vi "Report.WR.vi"(0 "Report Path":path=path "C:/Documents and Settings/Administrator/桌面", 1 "TestTime":dbl, 2 "TestRecord":T2={"name_pf"="Product_name", "name_name_ean13"="input SN", "supplier_code"="", "date"="", "time"="", "operater_code"="0", "sw_code"="", "sw_ver"="V10", "test_type"="EOL", "spare"="", "jig_code"="T001", "total_qty"="0", "field_code"="", "test_time"="NA", "test_result"="NA", "serial_number"="input SN", "TestItem"=[]}, 4 "SN":string, 5 "Result":enum16{"PASS", "FAIL", "INT.", "TOUT"}(ring)=enum."FAIL", 6 "TestTime":T1) -> (7 "OK?":bool=TRUE, 8 "TestTime?":bool, 9 "FileName":string="C:\\Documents and Settings\\Administrator\\桌面\\report\\Product_name_T001_EOL_800324.txt")   [LabVIEW 2012, in "Lib_UEL.ATE.lvlib" / "Lib_Report.lvlib"]
uses:
  Lib_Report.lvlib
panel:
  out "SystemTime":string="20121102  17:33:22 "
  # "ChangeLog\n2014-6-19: 根据UD反馈，修改栏目对齐问题。"
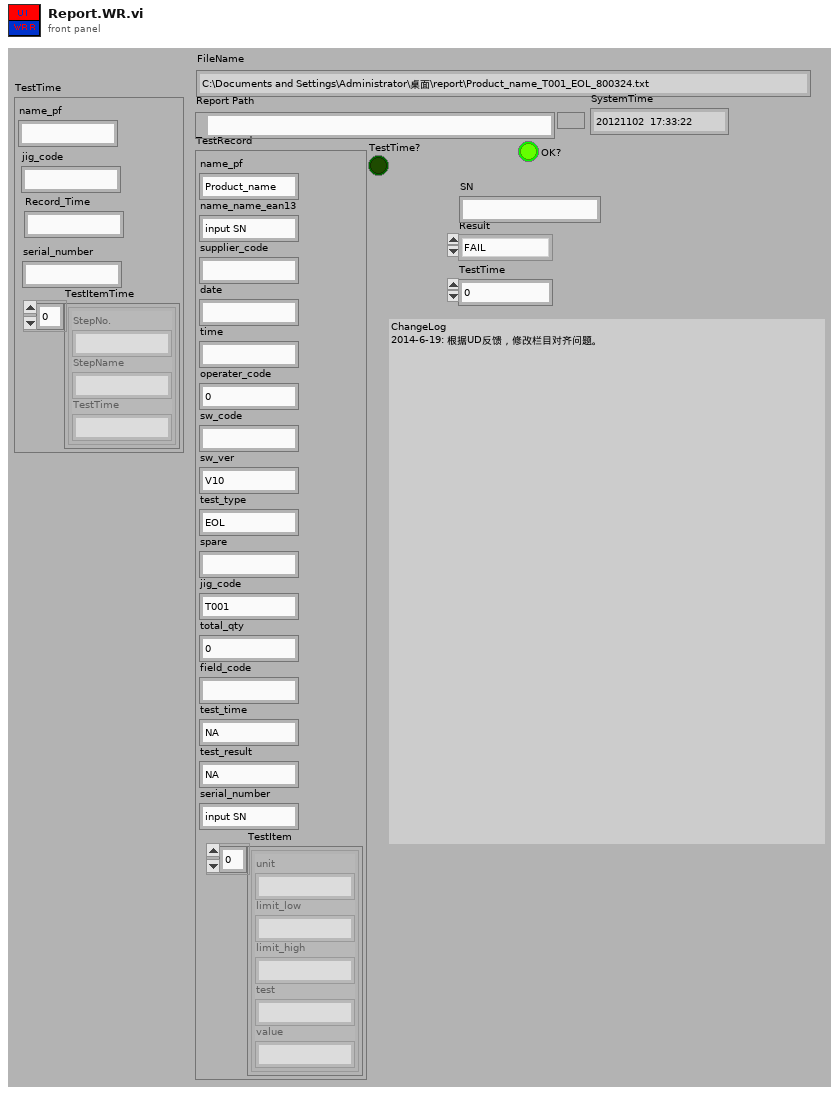
[diagram p1: front panel]
types:
  T1 = cluster{"name_pf":string, "jig_code":string, "Record_Time":string, "serial_number":string, "TestItemTime":cluster{"StepNo.":string, "StepName":string, "TestTime":string}[]}
  T2 = cluster{"name_pf":string, "name_name_ean13":string, "supplier_code":string, "date":string, "time":string, "operater_code":string, "sw_code":string, "sw_ver":string, "test_type":string, "spare":string, "jig_code":string, "total_qty":string, "field_code":string, "test_time":string, "test_result":string, "serial_number":string, "TestItem":cluster{"unit":string, "limit_low":string, "limit_high":string, "test":string, "value":string}[]}
  T3 = enum16{"open", "replace", "create", "open or create", "replace or create", "replace or create with confirmation"}
  T4 = cluster{"unit":string, "limit_low":string, "limit_high":string, "test":string, "value":string}[]
  T5 = cluster{"StepNo.":string, "StepName":string, "TestTime":string}[]
  T6 = cluster{"unit":string, "limit_low":string, "limit_high":string, "test":string, "value":string}
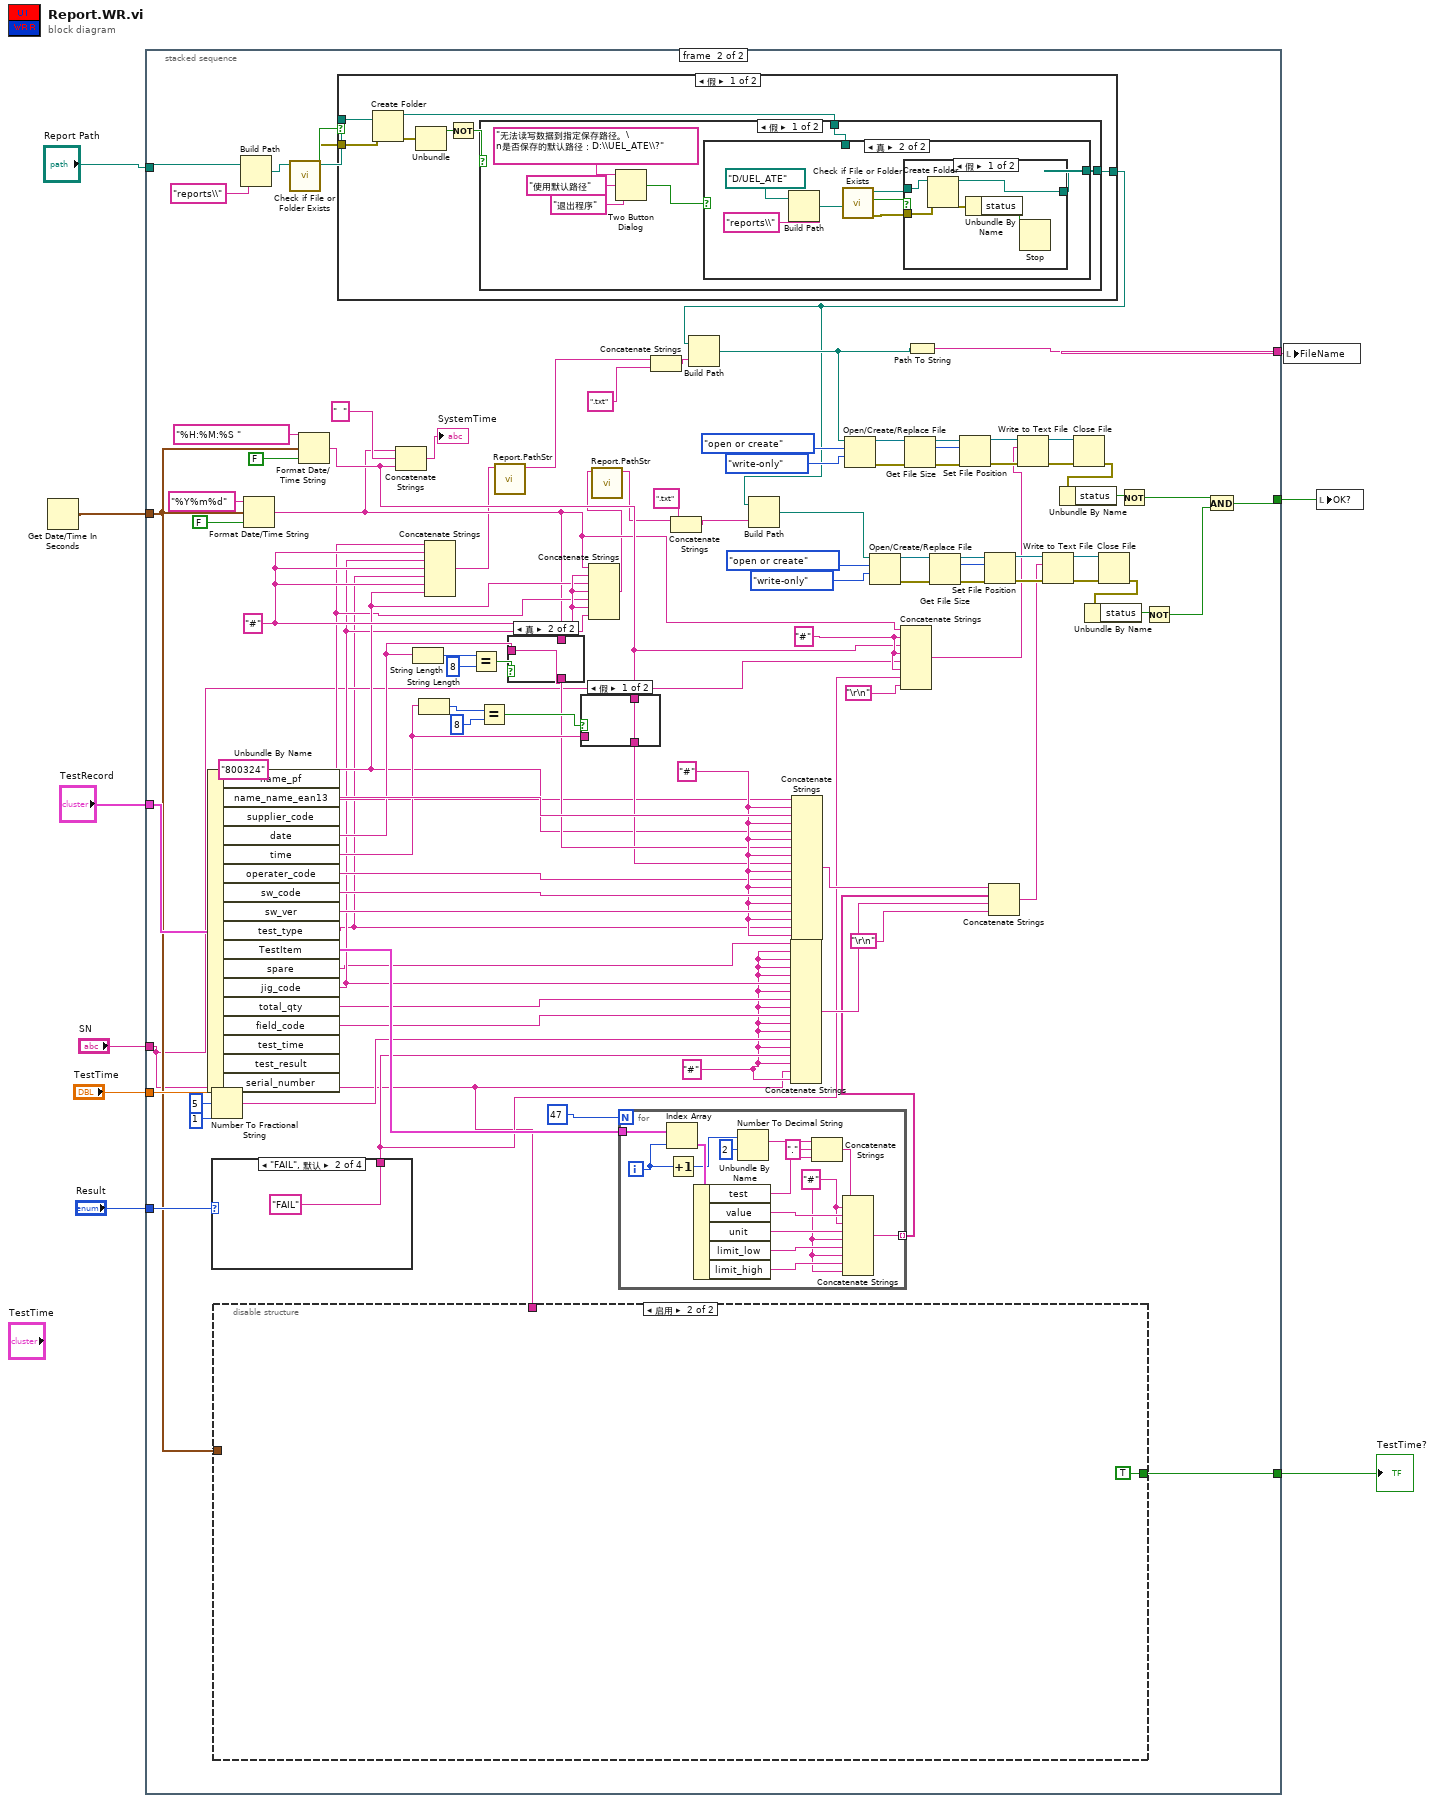
[diagram p0: block diagram]
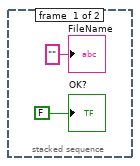
[diagram p2: hidden frame]
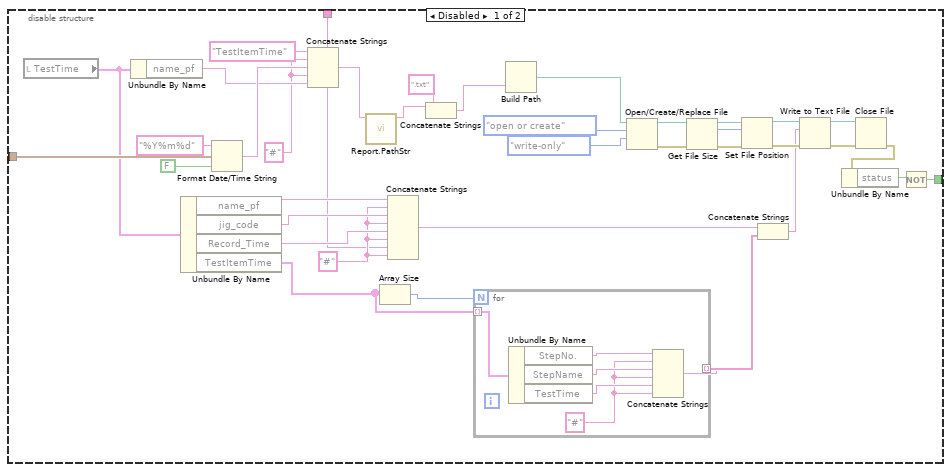
[diagram p3: hidden frame]
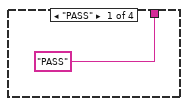
[diagram p4: hidden frame]
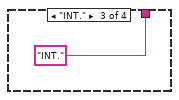
[diagram p5: hidden frame]
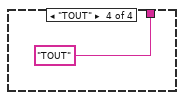
[diagram p6: hidden frame]
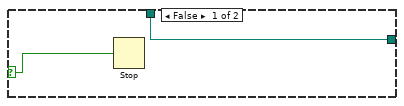
[diagram p9: hidden frame]
diagram:
  n1 = Get Date/Time In Seconds() -> (seconds since 1Jan1904=w8:timestamp)
  n2 = stacked-sequence {
    tunnel: "Report Path" -> [_ w21]
    tunnel: w8 -> [_ w15]
    tunnel: "TestRecord" -> [_ w101]
    tunnel: [_ w83] -> w6
    tunnel: [_ w29] -> w5
    tunnel: "Result" -> [_ w58]
    tunnel: "TestTime" -> [_ w57]
    tunnel: "SN" -> [_ w13]
    tunnel: [_ w14] -> w1
    frame #0 {
      "FileName" <- "" ("FileName")
      "OK?" <- FALSE ("OK?")
    }
    frame #1 {
      w33 = "#" ("字符串")
      w40 = "#" ("字符串")
      w39 = "800324" ("字符串")
      w17 = "#" ("字符串")
      w95 = "#" ("字符串")
      n3 = Unbundle By Name(w101) -> ("name_pf"=w38:string, "name_name_ean13"=w98:string, "date"=w64:string, "time"=w63:string, "operater_code"=w59:string, "sw_code"=w97:string, "sw_ver"=w96:string, "test_type"=w12:string, "TestItem"=w99:T4, "spare"=w20:string, "jig_code"=w37:string, "total_qty"=w94:string, "field_code"=w93:string)  [unwired: 4 out]
      n4 = Number To Fractional String(number=w57, width (-)=i16 5 ("宽度(-)"), precision (6)=i16 1 ("精度(6)")) -> (F-format string=w18:string)  [unwired: 1 in]
      n5 = case shown="\"FAIL\", 默认" w58 {
        tunnel: ["PASS" ("字符串") "FAIL" ("字符串") "INT." ("字符串") "TOUT" ("字符串")] -> w19
        frame "PASS" {
        }
        frame "FAIL", Default {
        }
        frame "INT." {
        }
        frame "TOUT" {
        }
      }
      n6 = disable-structure shown="启用" {
        disable-tunnel: w15 -> [w128 _]
        disable-tunnel: [w124 TRUE] -> w14
        disable-tunnel: w13 -> [w118 _]
        frame Disabled {
          w119 = "#" ("字符串")
          w112 = "#" ("字符串")
          n7 = local read "TestTime"() -> (w122:T1)
          n8 = Unbundle By Name(w122) -> ("name_pf"=w126:string)
          n9 = Unbundle By Name(w122) -> ("name_pf"=w123:string, "jig_code"=w121:string, "Record_Time"=w120:string, "TestItemTime"=w116:T5)
          n10 = Format Date/Time String(time format string (%c)="%Y%m%d" ("时间格式化字符串(%c)"), seconds (now)=w128, UTC format=FALSE ("UTC格式")) -> (date/time string=w127:string)
          n11 = Concatenate Strings("TestItemTime" ("字符串"), w112, w127, w112, w126) -> (w125:string)
          n12 = call "Report.PathStr.vi"("FilePath In"=w125) -> ("FilePath Out"=w132:string)  [unwired: 10 in]
          n13 = Array Size(array=w116) -> (size(s)=w117:i32)
          n14 = Concatenate Strings(w123, w119, w121, w119, w120, w119, w118, w119) -> (w115:string)
          n15 = Concatenate Strings(w132, ".txt" ("字符串")) -> (w131:string)
          n16 = for {
            N: w117 -> [_]
            tunnel: w116 -> [w152] mode=indexing
            tunnel: [w153] -> w114 mode=indexing
            w148 = "#" ("字符串")
            n17 = Unbundle By Name(w152) -> ("StepNo."=w151:string, "StepName"=w150:string, "TestTime"=w149:string)
            n18 = Concatenate Strings(w151, w148, w150, w148, w149, w148) -> (w153:string)
          }
          n19 = Build Path(name or relative path=w131) -> (appended path=w147:path)  [unwired: 1 in]
          n20 = Open/Create/Replace File(file path (use dialog)=w147, operation (0:open)=T3."open or create" ("运行（0:打开）"), access (0:read/write)=enum16{"read/write", "read-only", "write-only"}."write-only" ("访问（0:读取/写入）")) -> (refnum out=w142:refnum<file>, error out=w141:errorcluster)  [unwired: 3 in, 1 out]
          n21 = Get File Size(file=w142, error in=w141) -> (refnum out=w139:refnum<file>, size (in bytes)=w136:i64, 0:w138:errorcluster)
          n22 = Set File Position(offset (in bytes) (0)=w136, refnum=w139, error in=w138) -> (refnum out=w137:refnum<file>, error out=w140:errorcluster)  [unwired: 1 in]
          n23 = Concatenate Strings(w115, w114) -> (w113:string)
          n24 = Write to Text File(file (use dialog)=w137, text=w113, error in=w140) -> (refnum out=w144:refnum<file>, error out=w143:errorcluster)  [unwired: 1 in, 1 out]
          n25 = Close File(refnum=w144, error in=w143) -> (error out=w135:errorcluster)  [unwired: 1 out]
          n26 = Unbundle By Name(w135) -> ("status"=w134:bool)
          n27 = Not(x=w134) -> (.not. x?=w124:bool)
        }
        frame Enabled {
        }
      }
      n28 = Build Path(base path=w21, name or relative path="reports\\" ("名称或相对路径")) -> (appended path=w102:path)
      n29 = Format Date/Time String(time format string (%c)="%Y%m%d" ("时间格式化字符串(%c)"), seconds (now)=w15, UTC format=FALSE ("UTC格式")) -> (date/time string=w31:string)
      n30 = call <vilib>:"Check if File or Folder Exists.vi"("path"=w102) -> ("error out"=w107:errorcluster, "file or folder exists?"=w109:bool, "dup path"=w108:path)  [unwired: 8 in]
      n31 = Format Date/Time String(time format string (%c)="%H:%M:%S " ("时间格式化字符串(%c)"), seconds (now)=w15, UTC format=FALSE ("UTC格式")) -> (date/time string=w32:string)
      n32 = case shown="假" w109 {
        tunnel: [w179 w207] -> w35
        tunnel: w108 -> [w183 w207]
        tunnel: w107 -> [w184 _]
        frame False {
          n33 = Create Folder(path (use dialog)=w183, error in=w184) -> (created path=w178:path, error out=w182:errorcluster)  [unwired: 1 in, 1 out]
          n34 = Unbundle(w182) -> ("status"=w181:bool)  [unwired: 2 out]
          n35 = Not(x=w181) -> (.not. x?=w180:bool)
          n36 = case shown="假" w180 {
            tunnel: [w189 w206] -> w179
            tunnel: w178 -> [w188 w206]
            frame False {
              n37 = Two Button Dialog(message="无法读写数据到指定保存路径。\n是否保存的默认路径：D:\\UEL_ATE\\?" ("消息"), 1:"退出程序" ("F按钮名称（“取消”）"), 2:"使用默认路径" ("T按钮名称（“确定”）")) -> (T button?=w187:bool)
              n38 = case shown="真" w187 {
                selector: w187 -> [w191 _]
                tunnel: [w192 w193] -> w189
                tunnel: w188 -> [w192 _]
                frame False {
                  n39 = Stop(stop? (T)=w191) -> ()
                }
                frame True {
                  n40 = Build Path(base path=path "D:/UEL_ATE" ("基路径"), name or relative path="reports\\" ("名称或相对路径")) -> (appended path=w197:path)
                  n41 = call <vilib>:"Check if File or Folder Exists.vi"("path"=w197) -> ("error out"=w195:errorcluster, "file or folder exists?"=w194:bool, "dup path"=w196:path)  [unwired: 8 in]
                  n42 = case shown="假" w194 {
                    tunnel: w196 -> [w202 w205]
                    tunnel: [w204 w205] -> w193
                    tunnel: w195 -> [w203 _]
                    frame False {
                      n43 = Create Folder(path (use dialog)=w202, error in=w203) -> (created path=w204:path, error out=w201:errorcluster)  [unwired: 1 in, 1 out]
                      n44 = Unbundle By Name(w201) -> ("status"=w200:bool)
                      n45 = Stop(stop? (T)=w200) -> ()
                    }
                    frame True {
                    }
                  }
                }
              }
            }
            frame True {
            }
          }
        }
        frame True {
        }
      }
      n46 = Concatenate Strings(w31, "  " ("字符串"), w32) -> (→"SystemTime":string)
      n47 = String Length(string=w64) -> (length=w70:i32)
      n48 = String Length(string=w63) -> (length=w67:i32)
      n49 = Concatenate Strings(w38, w40, w37, w40, w12, w40, w39) -> (w26:string)
      n50 = Equal?(x=w70, y=8) -> (x = y?=w68:bool)
      n51 = Equal?(x=w67, y=8) -> (x = y?=w65:bool)
      n52 = call "Report.PathStr.vi"("FilePath In"=w26) -> ("FilePath Out"=w25:string)  [unwired: 10 in]
      n53 = case shown="真" w68 {
        tunnel: [w161 w162] -> w61
        tunnel: w31 -> [w161 _]
        tunnel: w64 -> [_ w162]
        frame False {
        }
        frame True {
        }
      }
      n54 = case shown="假" w65 {
        tunnel: [w159 w160] -> w60
        tunnel: w32 -> [w159 _]
        tunnel: w63 -> [_ w160]
        frame False {
        }
        frame True {
        }
      }
      n55 = Concatenate Strings(w31, w40, w39, w40, w38, w40, w37) -> (w24:string)
      n56 = call "Report.PathStr.vi"("FilePath In"=w24) -> ("FilePath Out"=w22:string)  [unwired: 10 in]
      n57 = for {
        N: 47 -> [_]
        tunnel: w99 -> [w177]
        tunnel: [w171] -> w82 mode=indexing
        i -> [w167]
        w169 = "#" ("字符串")
        n58 = Index Array(array=w177, index=w167) -> (element=w176:T6)
        n59 = Increment(x=w167) -> (x+1=w166:i32)
        n60 = Unbundle By Name(w176) -> ("test"=w165:string, "value"=w175:string, "unit"=w174:string, "limit_low"=w173:string, "limit_high"=w172:string)
        n61 = Number To Decimal String(number=w166, width (-)=i16 2 ("宽度(-)")) -> (decimal integer string=w168:string)
        n62 = Concatenate Strings(w168, "." ("字符串"), w165) -> (w163:string)
        n63 = Concatenate Strings(w163, w169, w175, w169, w174, w169, w173, w169, w172, w169) -> (w171:string)
      }
      n64 = Concatenate Strings(w25, ".txt" ("字符串")) -> (w87:string)
      n65 = Concatenate Strings(w22, ".txt" ("字符串")) -> (w36:string)
      n66 = Build Path(base path=w35, name or relative path=w87) -> (appended path=w84:path)
      n67 = Build Path(base path=w35, name or relative path=w36) -> (appended path=w16:path)
      n68 = Concatenate Strings(w20, w17, w17, w17, w17, w37, w17, w94, w17, w93, w17, w17, w18, w17, w19, w17, w13, w17) -> (w91:string)
      n69 = Concatenate Strings(w38, w95, w98, w95, w39, w95, w61, w95, w60, w95, w59, w95, w97, w95, w96, w95, w12, w95) -> (w92:string)
      n70 = Open/Create/Replace File(file path (use dialog)=w84, operation (0:open)=T3."open or create" ("运行（0:打开）"), access (0:read/write)=enum16{"read/write", "read-only", "write-only"}."write-only" ("访问（0:读取/写入）")) -> (refnum out=w81:refnum<file>, error out=w80:errorcluster)  [unwired: 3 in, 1 out]
      n71 = Open/Create/Replace File(file path (use dialog)=w16, operation (0:open)=T3."open or create" ("运行（0:打开）"), access (0:read/write)=enum16{"read/write", "read-only", "write-only"}."write-only" ("访问（0:读取/写入）")) -> (refnum out=w46:refnum<file>, error out=w47:errorcluster)  [unwired: 3 in, 1 out]
      n72 = Concatenate Strings(w31, w33, w32, w33, w13, w33, w19, "\r\n") -> (w34:string)
      n73 = Get File Size(file=w81, error in=w80) -> (refnum out=w78:refnum<file>, size (in bytes)=w75:i64, 0:w77:errorcluster)
      n74 = Path To String(path=w84) -> (string=w83:string)
      n75 = Get File Size(file=w46, error in=w47) -> (refnum out=w49:refnum<file>, size (in bytes)=w52:i64, 0:w50:errorcluster)
      n76 = Set File Position(offset (in bytes) (0)=w75, refnum=w78, error in=w77) -> (refnum out=w76:refnum<file>, error out=w79:errorcluster)  [unwired: 1 in]
      n77 = Set File Position(offset (in bytes) (0)=w52, refnum=w49, error in=w50) -> (refnum out=w51:refnum<file>, error out=w48:errorcluster)  [unwired: 1 in]
      n78 = Concatenate Strings(w92, w82, w91, "\r\n") -> (w41:string)
      n79 = Write to Text File(file (use dialog)=w76, text=w34, error in=w79) -> (refnum out=w86:refnum<file>, error out=w85:errorcluster)  [unwired: 1 in, 1 out]
      n80 = Write to Text File(file (use dialog)=w51, text=w41, error in=w48) -> (refnum out=w44:refnum<file>, error out=w45:errorcluster)  [unwired: 1 in, 1 out]
      n81 = Close File(refnum=w86, error in=w85) -> (error out=w73:errorcluster)  [unwired: 1 out]
      n82 = Unbundle By Name(w73) -> ("status"=w72:bool)
      n83 = Close File(refnum=w44, error in=w45) -> (error out=w53:errorcluster)  [unwired: 1 out]
      n84 = Unbundle By Name(w53) -> ("status"=w54:bool)
      n85 = Not(x=w72) -> (.not. x?=w28:bool)
      n86 = Not(x=w54) -> (.not. x?=w27:bool)
      n87 = And(x=w28, y=w27) -> (x .and. y?=w29:bool)
    }
  }
  "TestTime?" <- w1
  n88 = local write "FileName"(w6) -> ()
  n89 = local write "OK?"(w5) -> ()
